vi "Odour_bottle_VI.vi"() -> ()   [LabVIEW 2016]
panel:
  in  "Name":string="BOTTLE 1"
  in  "VPs":cluster{"X":dbl, "Y":dbl}[](graph)
  in  "Chemicals":i32[](listbox)
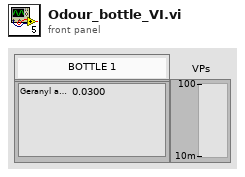
[diagram p1: front panel]
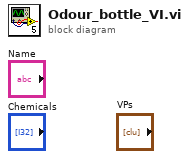
[diagram p0: block diagram]
diagram:
